vi "data test.vi"() -> ()   [LabVIEW 2020]
panel:
  out "Array 2":i32[][](array[numeric])
  out "Array":i32[](array[numeric])
  out "Waveform Chart":i32(graph)
  in  "stop":bool
  out "read buffer":string
  out "Device Name 2":string[](array[string])=["", "", "", "", "\n"]
  out "Num Dev 2":u32
  out "Device Address 2":refnum<visa-resource-name>[](array[refnum])
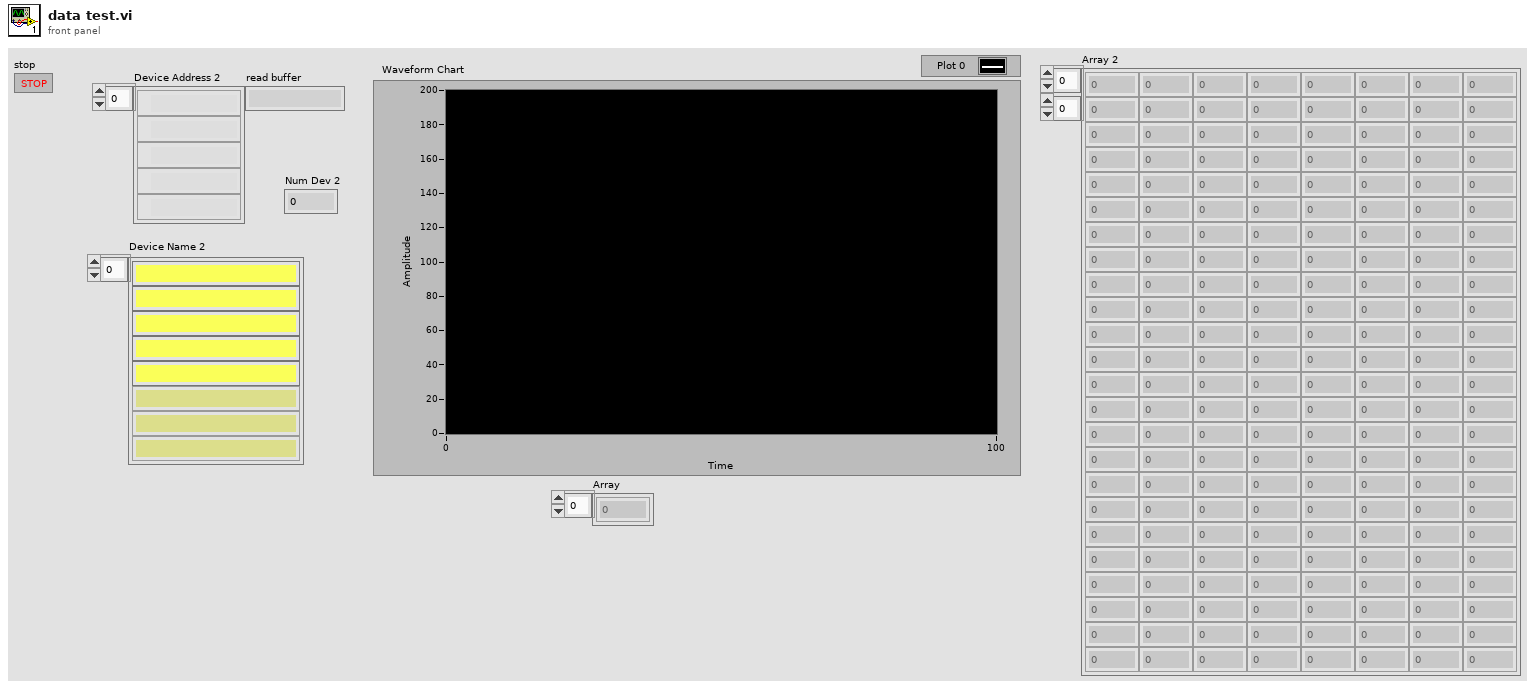
[diagram p1: front panel]
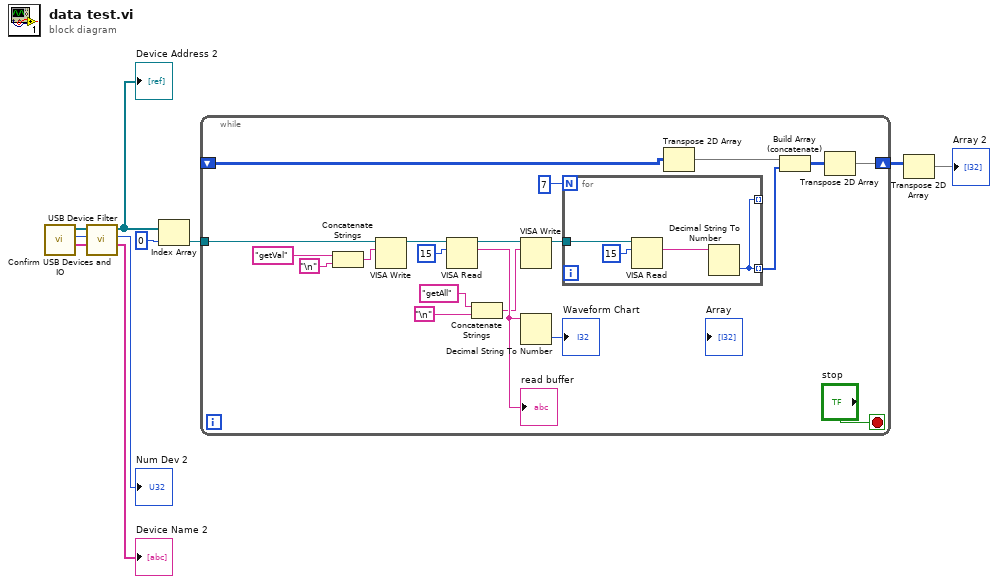
[diagram p0: block diagram]
diagram:
  n1 = call "Confirm USB Devices and IO.vi"() -> ("Device Name"=w10:string[], "Num Dev"=w9:u32, "Device Address"=w8:refnum<visa-resource-name>[])  [unwired: 9 in]
  n2 = call "USB Device Filter.vi"("Device Name"=w10, "Num Dev"=w9, "Device Address"=w8) -> ("Device Name 2"=→"Device Name 2":string[], "Num Dev 2"=→"Num Dev 2":u32, "Device Address 2"=w5:refnum<visa-resource-name>[])  [unwired: 6 in]
  "Device Address 2" <- w5
  n3 = Index Array(array=w5, index=0) -> (element=w3:refnum<visa-resource-name>)
  n4 = while {
    tunnel: w3 -> [w26]
    shift-right: [w11] -> w2
    shift-left: _ -> [w14]
    stop <- "stop" stop-if-true
    n5 = Concatenate Strings("getVal", "\n") -> (w29:string)
    n6 = VISA Write(VISA resource name=w26, write buffer=w29) -> (VISA resource name out=w25:refnum<visa-resource-name>)  [unwired: 1 in, 2 out]
    n7 = VISA Read(VISA resource name=w25, byte count=u32 15) -> (VISA resource name out=w17:refnum<visa-resource-name>, read buffer=w23:string)  [unwired: 1 in, 2 out]
    "read buffer" <- w23
    n8 = Concatenate Strings("getAll", "\n") -> (w20:string)
    n9 = VISA Write(VISA resource name=w17, write buffer=w20) -> (VISA resource name out=w18:refnum<visa-resource-name>)  [unwired: 1 in, 2 out]
    n10 = Decimal String To Number(string=w23) -> (number=→"Waveform Chart":i32)  [unwired: 2 in, 1 out]
    n11 = for {
      N: 7 -> [_]
      tunnel: w18 -> [w33]
      tunnel: [w31] -> _ mode=indexing
      tunnel: [w31] -> w13 mode=indexing
      n12 = VISA Read(VISA resource name=w33, byte count=u32 15) -> (read buffer=w32:string)  [unwired: 1 in, 3 out]
      n13 = Decimal String To Number(string=w32) -> (number=w31:i32)  [unwired: 2 in, 1 out]
    }
    n14 = Transpose 2D Array(2D array=w14) -> (transposed array=w15:i32[][])
    n15 = Build Array (concatenate)(w15, w13) -> (w12:i32[][])
    n16 = Transpose 2D Array(2D array=w12) -> (transposed array=w11:i32[][])
  }
  n17 = Transpose 2D Array(2D array=w2) -> (transposed array=→"Array 2":i32[][])
